vi "Set UI Control Value.vi"(8 "error in (no error)":errorcluster, 10 "VI Ref":refnum<vi>, 11 "Double Parameter in":refnum<class "Double Parameter.lvclass">) -> (0 "error out":errorcluster, 3 "Double Parameter out":refnum<class "Double Parameter.lvclass">)   [LabVIEW 2016, in "CD Parameter Manager API.lvlib" / "Double Parameter.lvclass"]
uses:
  Double Parameter.lvclass
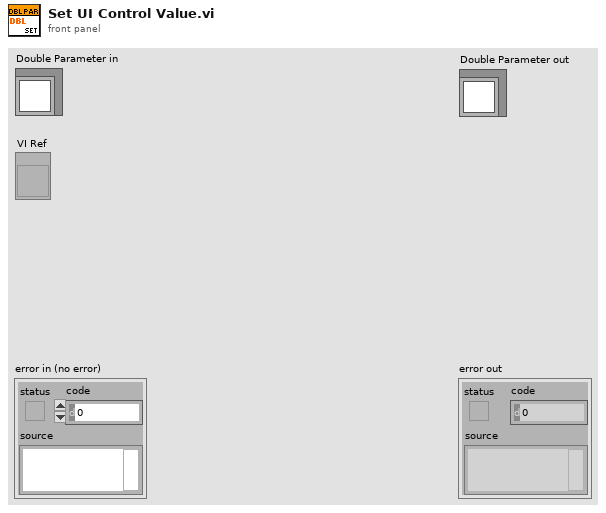
[diagram p1: front panel]
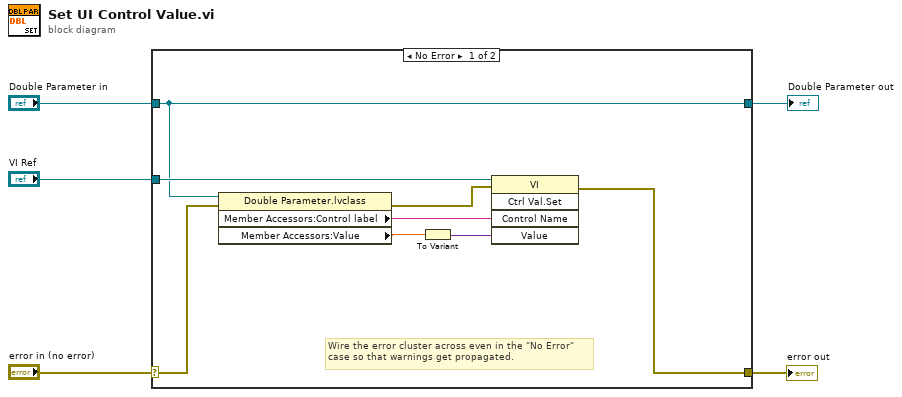
[diagram p0: block diagram]
diagram:
  n1 = case shown="No Error" "error in (no error)" {
    selector: "error in (no error)" -> [w7 w15]
    tunnel: [w12 w15] -> w1
    tunnel: "VI Ref" -> [w11 _]
    tunnel: [w10 w14] -> w5
    tunnel: "Double Parameter in" -> [w10 w14]
    frame No Error {
      # "Wire the error cluster across even in the \"No Error\"\ncase so that warnings get propagated."
      n2 = property class="Double Parameter.lvclass"(reference=w10, error in=w7) -> (error out=w6:errorcluster, "Member Accessors:Control label"=w9:string, "Member Accessors:Value"=w8:dbl)  [unwired: 1 out]
      n3 = To Variant(anything=w8) -> (Variant=w13:variant)
      n4 = invoke class="VI" method="Ctrl Val.Set"(reference=w11, error in=w6, "Control Name"=w9, "Value"=w13) -> (error out=w12:errorcluster)  [unwired: 1 in, 4 out]
    }
    frame Error {
    }
  }
  "error out" <- w1
  "Double Parameter out" <- w5
